vi "LoadComicsFromFile.vi"(8 "error in (no error)":errorcluster, 11 "Comics in":refnum<class "Comics.lvclass">) -> (0 "error out":errorcluster, 3 "Comics out":refnum<class "Comics.lvclass">)   [LabVIEW 2022 SP3, in "Comics.lvclass"]
uses:
  Comics.lvclass
  Comics.lvclass/Comics.ctl
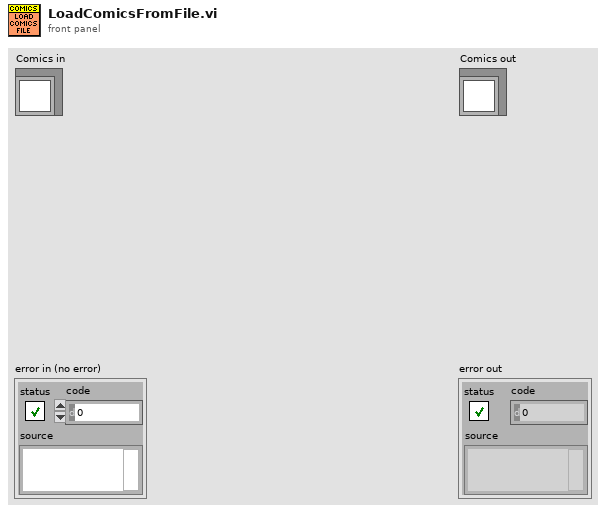
[diagram p1: front panel]
types:
  T1 = typedef "Comic.ctl" = cluster{"URL":string, "Series URL":string, "Series":string, "Volume":i32, "Issue":string, "Title":string, "Description":string, "Page Count":i32, "Cover Price":dbl, "UPC":string, "Characters":T2[], "Creators":T3[], "Main Cover URL":string, "Variant Covers":T4[], "DatePublished":timestamp}
  T2 = typedef "Character.ctl" = cluster{"Name":string, "Real-Name":string, "Universe":string, "URL":string}
  T3 = typedef "Creator.ctl" = cluster{"Name":string, "URL":string, "Creator Types":string[]}
  T4 = typedef "Variant.ctl" = cluster{"URL":string, "Description":string, "Cover URL":string}
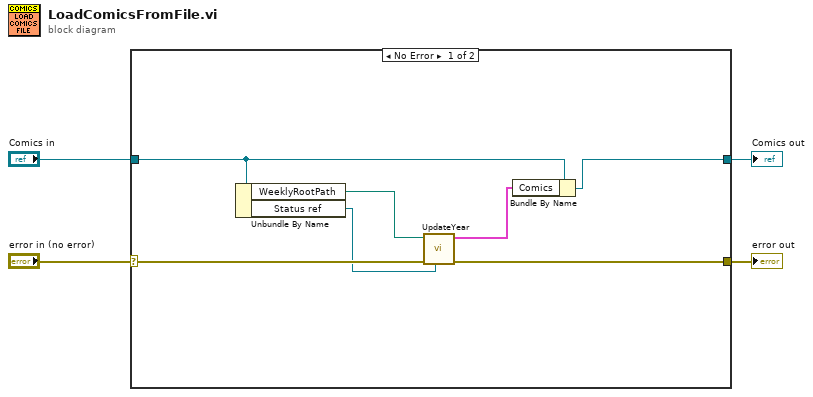
[diagram p0: block diagram]
diagram:
  n1 = case shown="No Error" "error in (no error)" {
    selector: "error in (no error)" -> [w11 w13]
    tunnel: [w10 w13] -> w3
    tunnel: [w5 w12] -> w1
    tunnel: "Comics in" -> [w7 w12]
    frame No Error {
      n2 = Unbundle By Name(w7) -> ("WeeklyRootPath"=w9:path, "Status ref"=w8:refnum<vi>)
      n3 = call "UpdateYear.vi"("Status ref"=w8, "error in"=w11, "Year Folder"=w9) -> ("error out"=w10:errorcluster, "Comics"=w6:T1[])  [unwired: 7 in]
      n4 = Bundle By Name(cluster=w7, "Comics"=w6) -> (w5:refnum<class "Comics.lvclass">)
    }
    frame Error {
    }
  }
  "error out" <- w3
  "Comics out" <- w1
